vi "PulsehistogramSimple3GHz_NI5771.vi"() -> ()   [LabVIEW 2012]
uses:
  <vilib>/Platform/TimedLoop/XDataNode/timing_clust.ctl
  <vilib>/Platform/TimedLoop/XDataNode/nitl_modes.ctl
  <vilib>/Platform/TimedLoop/XDataNode/wakeup.ctl
  <vilib>/rvi/eio/common/nirviEmuTemplateMethod_errors.vi
  <vilib>/rvi/Emulation/niFpgaSctlEmulationRegisterWithScheduler.vi
  <vilib>/rvi/DataTransferAndStorage/Container/Common/niFpgaContainerGetUniqueNameForEmu.vi
  <vilib>/rvi/FIFO/Fifo_Resource/nirvififoEmulationSetSize.vi
  <vilib>/rvi/errors/niFpgaSetErrorForExecOnDevCompSimple.vi
  <vilib>/rvi/eio/common/nirviEmuReportErrorAndStop.vi
  <vilib>/rvi/Emulation/niFpgaSctlEmulationFifoFullMgr.vi
  <vilib>/rvi/Emulation/niFpgaSctlEmulationResourceMgr.vi
  <vilib>/rvi/Emulation/niFpgaSctlEmulationScheduler.vi
  <vilib>/rvi/interface/RandomDataEmulation/nirviRandomDataFPGAFIFO.vi
  <vilib>/rvi/interface/RandomDataEmulation/niFpgaRandomDataHandleErrors.vi
  <vilib>/Platform/TimedLoop/XDataNode/XDataNode.xnode
  <vilib>/eio/EIONode/EIONode.xnode
  <vilib>/rvi/DataTransferAndStorage/Container/XNode/niFpgaContainer.xnode
  <vilib>/rvi/FIFO/Fifo_Resource/nirvififoEmulationWrite.vi
  <vilib>/rvi/FIFO/Fifo_Resource/nirvififoEmulationRead.vi
  <vilib>/rvi/interface/RandomDataEmulation/nirviRandomDataFpgaReadWriteTemplate.vi
  <vilib>/Platform/TimedLoop/XDataNode/XDNodeRunTimeDep.lvlib
panel:
  out "ToHostFIFO Overflow":bool caption="FIFO Overflow?"
  in  "Samples to acquire":u32
  out "InterloopFIFO overflow":bool
  out "IO Module\\AI Over Range":bool
  in  "User Command Commit":bool
  in  "User Command":u8
  out "User Command Idle":bool
  out "User Command Status":u8
  in  "User Data 0":u16
  in  "User Data 1":u8
  out "PLL Locked":bool
  out "User Error":bool
  out "Configured?":bool
  # "Analog acquisition 3 GHz (TIS mode)\nChannel 0 & trigger"
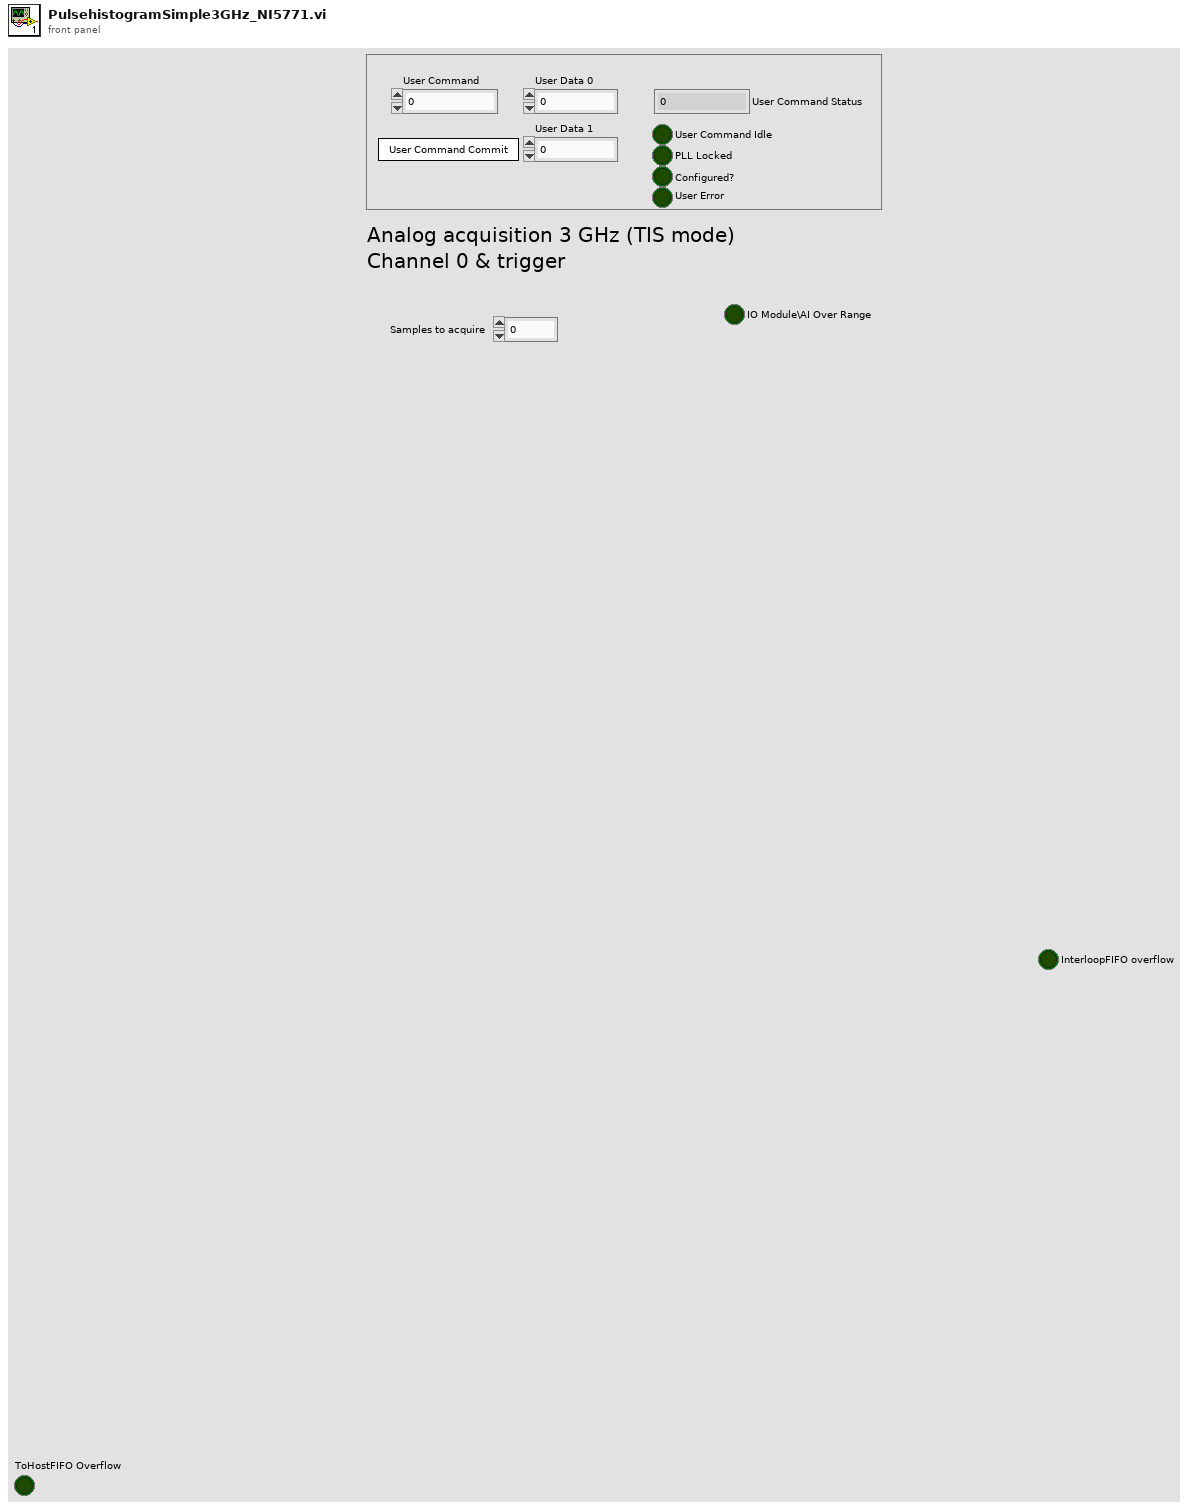
[diagram p1: front panel]
types:
  T1 = typedef "XDNodeRunTimeDep.lvlib/timing_clust.ctl" = cluster{"Expected End [f-1]":u64, "Actual End [f-1]":u64, "Finished Late? [f-1]":bool, "Expected End [i-1]":u64, "Actual End [i-1]":u64, "Finished Late? [i-1]":bool, "Expected Start [i]":u64, "Actual Start [i]":u64, "Expected Start [f]":u64, "Actual Start [f]":u64, "Source Name":string, "Structure Name":string, "Period":i64, "Deadline":i64, "Offset":i64, "Start":i64, "Priority":i32, "Timeout":i32, "Mode":T2, "Wakeup Reason":T3, "Error":errorcluster, "Source Type":string, "Secondary Source Type":string, "Global End Time":u64, "Global Start Time":u64, "Frame Duration":u64, "Iteration Duration":u64, "Assigned CPU":i32, "I/O Scan Engine Mode":u32}
  T2 = typedef "XDNodeRunTimeDep.lvlib/nitl_modes.ctl" = enum32{"No Change", "Process missed periods, maintain original phase", "Discard missed periods, maintain original phase", "Process missed periods, ignore original phase", "Discard missed periods, ignore original phase"}
  T3 = typedef "XDNodeRunTimeDep.lvlib/wakeup.ctl" = enum32{"Normal", "Aborted", "Asynchronous wakeup", "Timing source error", "Timed loop error", "Timeout"}
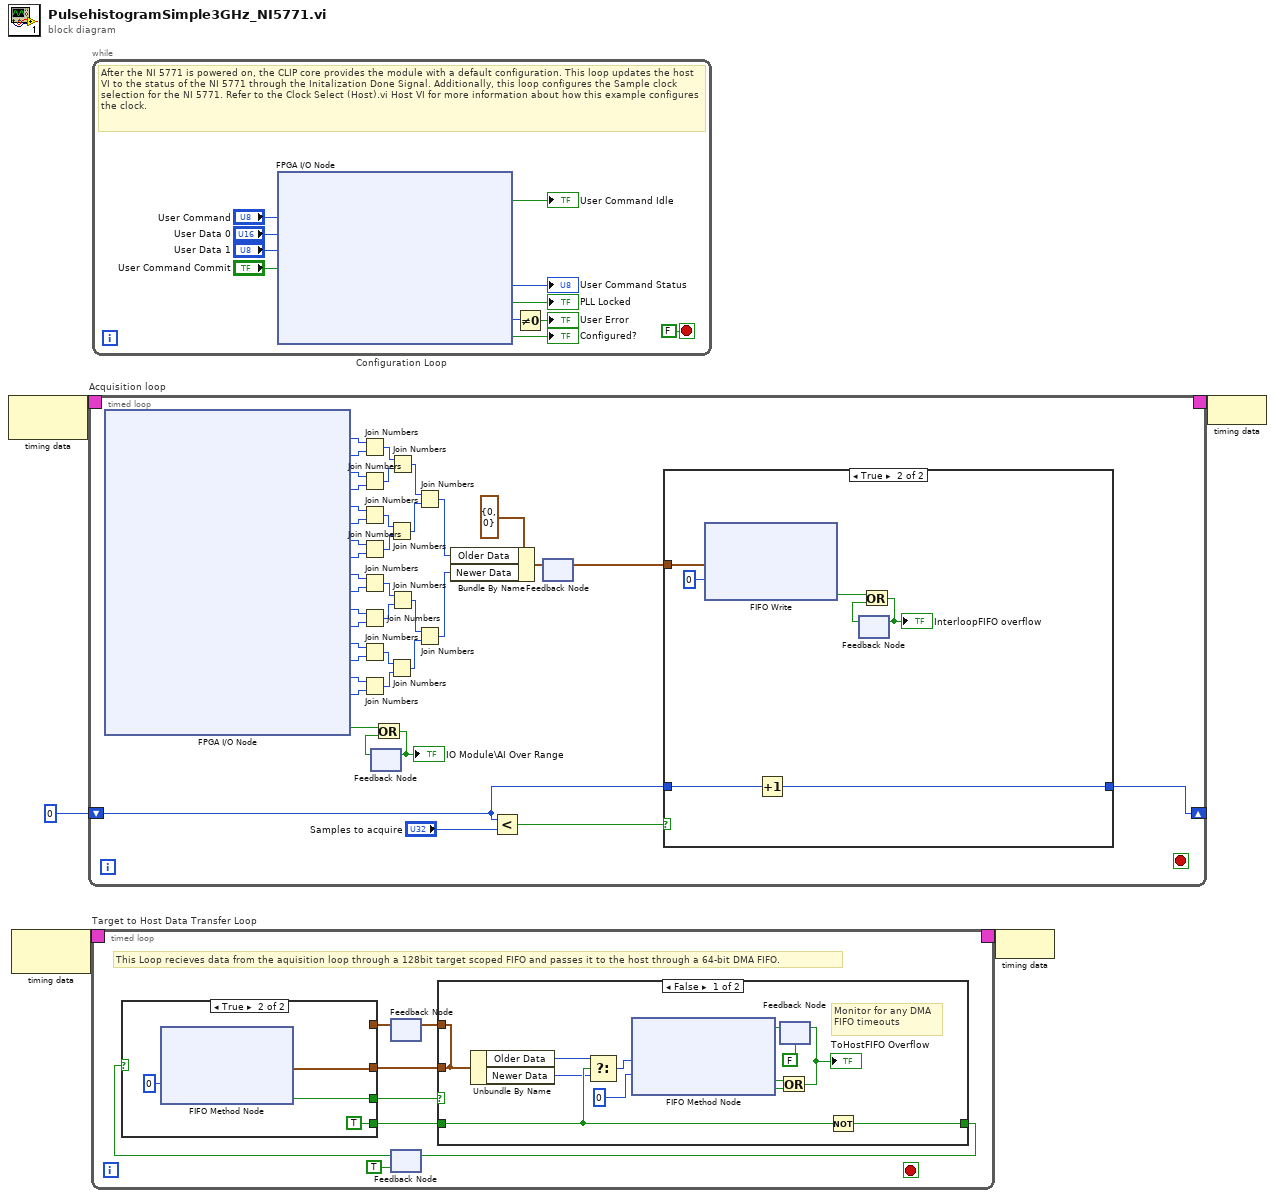
[diagram p0: block diagram]
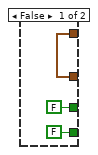
[diagram p2: hidden frame]
diagram:
  n1 = node-c288() -> (w5:T1)  [unwired: 1 in]
  n2 = node-c288() -> (w2:T1)  [unwired: 1 in]
  n3 = timed-loop "Acquisition loop" {
    timing: w5 -> [_]
    timing-out: [_] -> w4
    shift-right: [w6] -> _
    shift-left: u32 0 -> [w7]
    stop <- _ stop-if-true
    n4 = xnode "FPGA I/O Node"() -> ("IO Module\\AI 1 Data N-7"=w45:u8, "IO Module\\AI 0 Data N-7"=w44:u8, "IO Module\\AI 1 Data N-6"=w43:u8, "IO Module\\AI 0 Data N-6"=w38:u8, "IO Module\\AI 1 Data N-5"=w39:u8, "IO Module\\AI 0 Data N-5"=w42:u8, "IO Module\\AI 1 Data N-4"=w40:u8, "IO Module\\AI 0 Data N-4"=w41:u8, "IO Module\\AI 1 Data N-3"=w24:u8, "IO Module\\AI 0 Data N-3"=w23:u8, "IO Module\\AI 1 Data N-2"=w22:u8, "IO Module\\AI 0 Data N-2"=w21:u8, "IO Module\\AI 1 Data N-1"=w20:u8, "IO Module\\AI 0 Data N-1"=w19:u8, "IO Module\\AI 1 Data N"=w18:u8, "IO Module\\AI 0 Data N"=w25:u8, "IO Module\\AI Over Range"=w12:bool)  [unwired: 18 in, 19 out]
    n5 = Join Numbers(hi=w45, lo=w44) -> ((hi.lo)=w37:u16)
    n6 = Join Numbers(hi=w43, lo=w38) -> ((hi.lo)=w35:u16)
    n7 = Join Numbers(hi=w39, lo=w42) -> ((hi.lo)=w36:u16)
    n8 = Join Numbers(hi=w40, lo=w41) -> ((hi.lo)=w34:u16)
    n9 = Join Numbers(hi=w24, lo=w23) -> ((hi.lo)=w26:u16)
    n10 = Join Numbers(hi=w22, lo=w21) -> ((hi.lo)=w28:u16)
    n11 = Join Numbers(hi=w20, lo=w19) -> ((hi.lo)=w27:u16)
    n12 = Join Numbers(hi=w18, lo=w25) -> ((hi.lo)=w29:u16)
    n13 = feedback #1() -> (w11:bool)  [unwired: 1 in]
    n14 = Or(x=w12, y=w11) -> (x .or. y?=w10:bool)
    "IO Module\\AI Over Range" <- w10
    n15 = feedback-in #1(w10) -> ()
    n16 = Join Numbers(hi=w36, lo=w34) -> ((hi.lo)=w32:u32)
    n17 = Join Numbers(hi=w27, lo=w29) -> ((hi.lo)=w31:u32)
    n18 = Join Numbers(hi=w37, lo=w35) -> ((hi.lo)=w33:u32)
    n19 = Join Numbers(hi=w26, lo=w28) -> ((hi.lo)=w30:u32)
    n20 = Join Numbers(hi=w33, lo=w32) -> ((hi.lo)=w15:u64)
    n21 = Join Numbers(hi=w30, lo=w31) -> ((hi.lo)=w14:u64)
    n22 = Bundle By Name(cluster=cluster{"Older Data":u64, "Newer Data":u64} {"Older Data"=0, "Newer Data"=0} ("Element"), "Older Data"=w15, "Newer Data"=w14) -> (w16:cluster{"Older Data":u64, "Newer Data":u64})
    n23 = Less?(x=w7, y="Samples to acquire") -> (x < y?=w8:bool)
    n24 = feedback #2() -> (w13:cluster{"Older Data":u64, "Newer Data":u64})  [unwired: 1 in]
    n25 = feedback-in #2(w16) -> ()
    n26 = case shown="True" w8 {
      tunnel: w13 -> [_ w53]
      tunnel: w7 -> [w46 w49]
      tunnel: [w46 w48] -> w6
      frame False {
      }
      frame True {
        n27 = xnode ("FIFO Write")("Element"=w53, "Timeout"=0) -> ("Timed Out?"=w51:bool)  [unwired: 1 in, 1 out]
        n28 = Increment(x=w49) -> (x+1=w48:u32)
        n29 = feedback #3() -> (w50:bool)  [unwired: 1 in]
        n30 = Or(x=w51, y=w50) -> (x .or. y?=w52:bool)
        "InterloopFIFO overflow" <- w52
        n31 = feedback-in #3(w52) -> ()
      }
    }
  }
  n32 = timed-loop "Target to Host Data Transfer Loop" {
    timing: w2 -> [_]
    timing-out: [_] -> w1
    stop <- _ stop-if-true
    # "This Loop recieves data from the aquisition loop through a 128bit target scoped FIFO and passes it to the host through a 64-bit DMA FIFO."
    n33 = feedback #4() -> (w60:cluster{"Older Data":u64, "Newer Data":u64})  [unwired: 1 in]
    n34 = feedback #5(TRUE ("Timed Out?")) -> (w61:bool)
    n35 = case shown="True" w61 {
      tunnel: [w64 w67] -> w58
      tunnel: [FALSE ("Timed Out?") w68] -> w57
      tunnel: [FALSE ("Timed Out?") TRUE ("Timed Out?")] -> w56
      tunnel: w60 -> [w64 _]
      frame False {
      }
      frame True {
        n36 = xnode ("FIFO Method Node")("Timeout"=0) -> ("Element"=w67:cluster{"Older Data":u64, "Newer Data":u64}, "Timed Out?"=w68:bool)  [unwired: 1 in, 1 out]
      }
    }
    n37 = case shown="False" w57 {
      tunnel: [w76 w83] -> w62
      tunnel: w56 -> [w77 w83]
      tunnel: w58 -> [w75 w82]
      tunnel: [w75 w82] -> w59
      frame False {
        # "Monitor for any DMA FIFO timeouts"
        n38 = Unbundle By Name(w75) -> ("Older Data"=w78:u64, "Newer Data"=w71:u64)
        n39 = Select(t=w78, s=w77, f=w71) -> (s? t:f=w73:u64)
        n40 = xnode ("FIFO Method Node")("Element"=w73, "Timeout"=0) -> ("Timed Out?"=w74:bool)  [unwired: 1 in, 1 out]
        n41 = feedback #6(FALSE) -> (w81:bool)
        n42 = Or(x=w81, y=w74) -> (x .or. y?=w79:bool)
        "ToHostFIFO Overflow" <- w79
        n43 = feedback-in #6(w79) -> ()
        n44 = Not(x=w77) -> (.not. x?=w76:bool)
      }
      frame True {
      }
    }
    n45 = feedback-in #4(w59) -> ()
    n46 = feedback-in #5(w62) -> ()
  }
  n47 = while "Configuration Loop" {
    stop <- FALSE stop-if-true
    # "After the NI 5771 is powered on, the CLIP core provides the module with a default configuration. This loop updates the host VI to the status of the NI 5771 through the Initalization Done Signal. Additionally, this loop configures the Sample clock selection for the NI 5771. Refer to the Clock Select (Host).vi Host VI for more information about how this example configures the clock."
    n48 = xnode "FPGA I/O Node"("IO Module\\User Command"="User Command", "IO Module\\User Data 0"="User Data 0", "IO Module\\User Data 1"="User Data 1", "IO Module\\User Command Commit"="User Command Commit") -> ("IO Module\\User Command Idle"=→"User Command Idle":bool, "IO Module\\User Command Status"=→"User Command Status":u8, "IO Module\\PLL Locked"=→"PLL Locked":bool, "IO Module\\User Error"=w89:u8, "IO Module\\Initialization Done"=→"Configured?":bool)  [unwired: 9 in, 9 out]
    n49 = Not Equal To 0?(x=w89) -> (x != 0?=→"User Error":bool)
  }
  n50 = node-c288(w1) -> ()
  n51 = node-c288(w4) -> ()
